vi "Test.Python.vi"() -> ()   [LabVIEW 2014]
uses:
  python27.dll
panel:
  in  "Script":path=path "Test.py"
  in  "Test":bool caption="stop"
  in  "Content":string
  in  "Path":path
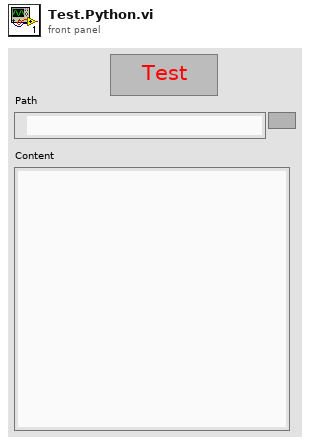
[diagram p1: front panel]
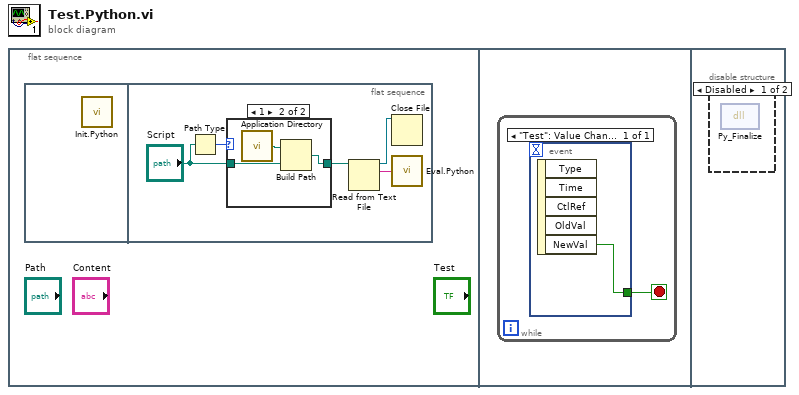
[diagram p0: block diagram]
diagram:
  n1 = flat-sequence {
    frame #0 {
      n2 = flat-sequence {
        frame #0 {
          n3 = call "Init.Python.vi"() -> ()  [unwired: 1 in]
        }
        frame #1 {
          n4 = Path Type(1:"Script") -> (0:w2:i16)
          n5 = case shown="1" w2 {
            tunnel: "Script" -> [w6 w8]
            tunnel: [w6 w7] -> w1
            frame 0, Default {
            }
            frame 1 {
              n6 = call <vilib>:"Application Directory.vi"() -> ("Application Directory"=w9:path)
              n7 = Build Path(base path=w9, name or relative path=w8) -> (appended path=w7:path)
            }
          }
          n8 = Read from Text File(file (use dialog)=w1) -> (refnum out=w5:refnum<file>, text=w4:string)  [unwired: 3 in, 2 out]
          n9 = Close File(refnum=w5) -> ()  [unwired: 1 in, 2 out]
          n10 = call "Eval.Python.vi"("input"=w4) -> ()
        }
      }
    }
    frame #1 {
      n11 = while {
        stop <- w10 stop-if-true
        n12 = event shown="[0] \"Test\": Value Change" {
          selector: _ -> [_]
          dyn-events: _ -> [_]
          timeout: _ -> [_]
          tunnel: [w11] -> w10
          event "Test": Value Change {
            n13 = event-data() -> ("NewVal"=w11:bool)  [unwired: 1 in, 4 out]
          }
        }
      }
    }
    frame #2 {
      n14 = disable-structure shown="Disabled" {
        frame Disabled {
          n15 = dll-call lib="python27.dll" fn="Py_Finalize"() -> ()  [unwired: 4 in, 2 out]
        }
        frame Enabled {
        }
      }
    }
  }
